vi "数据合并.vi"(10 "数值输入":dbl, 11 "数值 3":dbl) -> (3 "字符串":string)   [LabVIEW 2016]
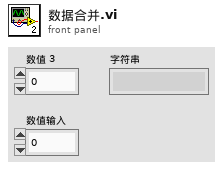
[diagram p1: front panel]
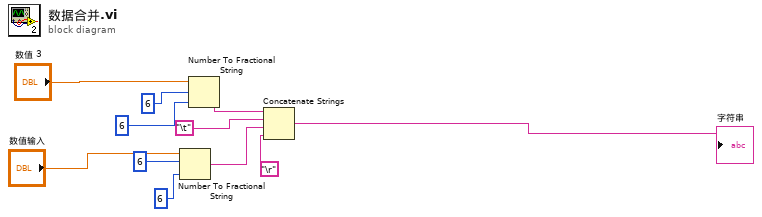
[diagram p0: block diagram]
diagram:
  n1 = Number To Fractional String(number="数值输入", width (-)=i16 6 ("宽度(-)"), precision (6)=i16 6 ("精度(6)")) -> (F-format string=w10:string)  [unwired: 1 in]
  n2 = Number To Fractional String(number="数值 3", width (-)=i16 6 ("宽度(-)"), precision (6)=i16 6 ("宽度(-)")) -> (F-format string=w2:string)  [unwired: 1 in]
  n3 = Concatenate Strings(w2, "\t", w10, "\r") -> (→"字符串":string)
